vi "imaqio_FindDevice.vi"(8 "error in (no error)":errorcluster, 11 "Resource In":string) -> (0 "error out":errorcluster, 2 "All Resources":string[](array[string]), 3 "Resource Out":string)   [LabVIEW 2017]
uses:
  <vilib>/LabVIEW Targets/FPGA/RIO/nirio_driverPrimitives.llb/_nirio_device_attributes.ctl
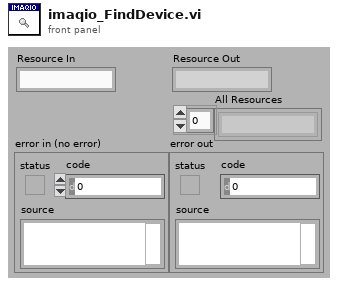
[diagram p1: front panel]
types:
  T1 = typedef "_nirio_device_attributes.ctl" = enum32{"kRioInitialized", "kRioInterfaceNum", "kRioProductNum", "kRioVendorNum", "kRioSerialNum", "kRioSignature", "kRioRsrcType", "kRioDeviceMgr", "kRioDefaultTimeout", "kRioLocalFifoRatio", "kRioBusNum", "kRioDeviceNum", "kRioFuncNum", "kRioRestrictedAccess", "kRioCurrentVersion", "kRioOldestCompatibleVersion", "kRioClientIsBigEndian", "kRioFpgaInterruptControlOffset", "kRioNumMemWindows", "kRioMemBaseBar0", "kRioMemBaseBar1", "kRioMemSizeBar0", "kRioMemSizeBar1", "kRioSessionState", "kRioPersonalityLockTimeout", "kRioAddressSpace", "Invalid", "kRioChassisNum", "kRioSlotNum", "kRioLocalFifoDefaultDepth", "kRioTriggerBusNum", "kRioTriggerReserveLine", "kRioTriggerUnreserveLine", "kRioTriggerReservedLines", "kRioIrqNodeReserve", "kRioFpgaInterruptEnable", "kRioIsItOkToDownload", "kRioFpgaResetOffset", "kRioFpgaResetWidthInBits", "kRioFpgaControlOffset", "kRioResetIfLastSession", "kRioHasDeviceAccess", "kRioBusInterfaceType", "kRioNumberOfDmaChannels", "kRioFpgaAddressSpaceOffset", "kRioBitstreamVersion", "kRioIsInAPciSlot", "kRioIsRio", "kRioIsFpgaProgrammed", "kRioFpgaGuid0", "kRioFpgaGuid1", "kRioFpgaGuid2", "kRioFpgaGuid3", "kRioFpgaDefaultSignatureOffset", "kRioFpgaDefaultResetOffset", "kRioFpgaDefaultResetSize", "kRioFpgaDefaultControlOffset", "kRioFpgaDefaultInterruptOffset", "kRioIsItOkToTalkToHardware", "kRioHasNoFPGASwitch", "kRioIrql", "kRioNumberOfDreqLines", "kRioFlashIoPortSize", "kRioFlashWindowNumber", "kRioFlashIoPortWindowSize", "kBoardFlashAutoLoadMode", "kRioHostInterfaceData", "kRioFlashWindowOffset", "kRioIsPciExpress", "kRioMemBaseBar", "kRioMemSizeBar", "kStc3P2PReaderDisabled", "kStc3P2PReaderEnabled"}
  T2 = typedef "_nirio_device_handleType.ctl" = u32
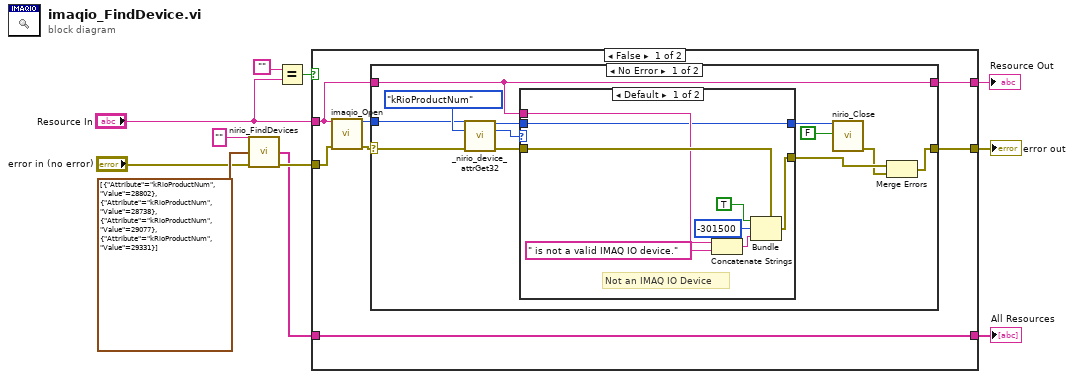
[diagram p0: block diagram]
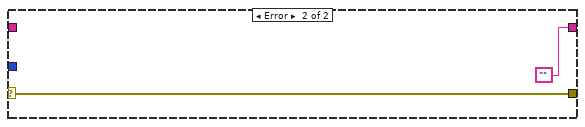
[diagram p3: hidden frame]
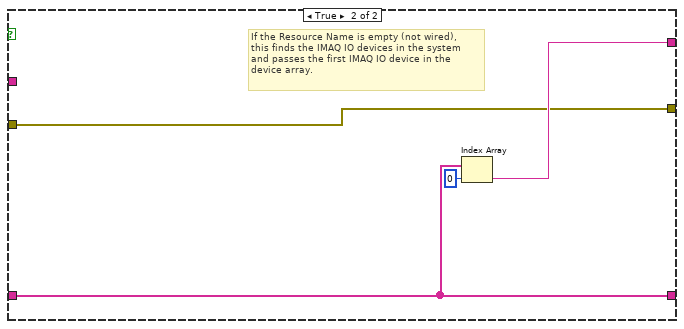
[diagram p4: hidden frame]
diagram:
  n1 = call <vilib>:"nirio_FindDevices.vi"("host URL (\"\": local)"="" ("host"), "Filter (empty: all devices)"=cluster{"Attribute":T1, "Value":u32}[] [{"Attribute"=enum."kRioProductNum", "Value"=28802}, {"Attribute"=enum."kRioProductNum", "Value"=28738}, {"Attribute"=enum."kRioProductNum", "Value"=29077}, {"Attribute"=enum."kRioProductNum", "Value"=29331}], "error in"="error in (no error)") -> ("devices"=w2:string[], "error out"=w3:errorcluster)  [unwired: 1 in, 10 out]
  n2 = Equal?(x="", y="Resource In") -> (x = y?=w10:bool)
  n3 = case shown="False" w10 {
    tunnel: w3 -> [w15 w44]
    tunnel: [w18 w44] -> w9
    tunnel: "Resource In" -> [w13 _]
    tunnel: [w14 w45] -> w7
    tunnel: [w12 w43] -> w1
    tunnel: w2 -> [w12 w43]
    frame False {
      n4 = call <vilib>:"imaqio_Open.vi"("Resource Name"=w13, "error in (no error)"=w15) -> ("Device Handle Out"=w16:T2, "error out"=w17:errorcluster)  [unwired: 1 in, 11 out]
      n5 = case shown="No Error" w17 {
        selector: w17 -> [w21 w42]
        tunnel: w16 -> [w25 _]
        tunnel: [w27 w42] -> w18
        tunnel: [w20 ""] -> w14
        tunnel: w13 -> [w20 _]
        frame No Error {
          n6 = call <vilib>:"_nirio_device_attrGet32.vi"("Device Handle In"=w25, "attribute"=_nirio_device_attributes."kRioProductNum", "error in"=w21) -> ("Device Handle Out"=w24:T2, "val"=w22:u32, "error out"=w23:errorcluster)  [unwired: 10 out]
          n7 = case shown="Default" w22 {
            tunnel: w24 -> [w31 w39]
            tunnel: w23 -> [w38 w40]
            tunnel: [w35 w40] -> w29
            tunnel: w20 -> [w32 _]
            tunnel: [w31 w39] -> w19
            frame Default {
              # "Not an IMAQ IO Device"
              n8 = Concatenate Strings(w32, " is not a valid IMAQ IO device." ("string")) -> (w36:string)
              n9 = Bundle(cluster=w38, "status"=TRUE, "code"=-301500, "source"=w36) -> (w35:errorcluster)
            }
            frame 28738, 28802, 29077, 29331 {
              # "Valid IMAQ IO Device"
            }
          }
          n10 = call <vilib>:"nirio_Close.vi"("handle in"=w19, "reset if last session (f)"=FALSE) -> ("error out"=w28:errorcluster)  [unwired: 1 in, 12 out]
          n11 = Merge Errors(w29, w28) -> (w27:errorcluster)
        }
        frame Error {
        }
      }
    }
    frame True {
      # "If the Resource Name is empty (not wired),\nthis finds the IMAQ IO devices in the system\nand passes the first IMAQ IO device in the \ndevice array."
      n12 = Index Array(array=w43, index=0) -> (element=w45:string)
    }
  }
  "error out" <- w9
  "Resource Out" <- w7
  "All Resources" <- w1
